vi "Read.Decrypt.7zPayload.vi"(8 "error in (no error)":errorcluster, 9 "Password":string="pw", 10 "File Folder Out":path, 11 "File Path":path) -> (0 "error out":errorcluster)   [LabVIEW 2020, in "PixPack.lvlib"]
uses:
  PixPack.lvlib
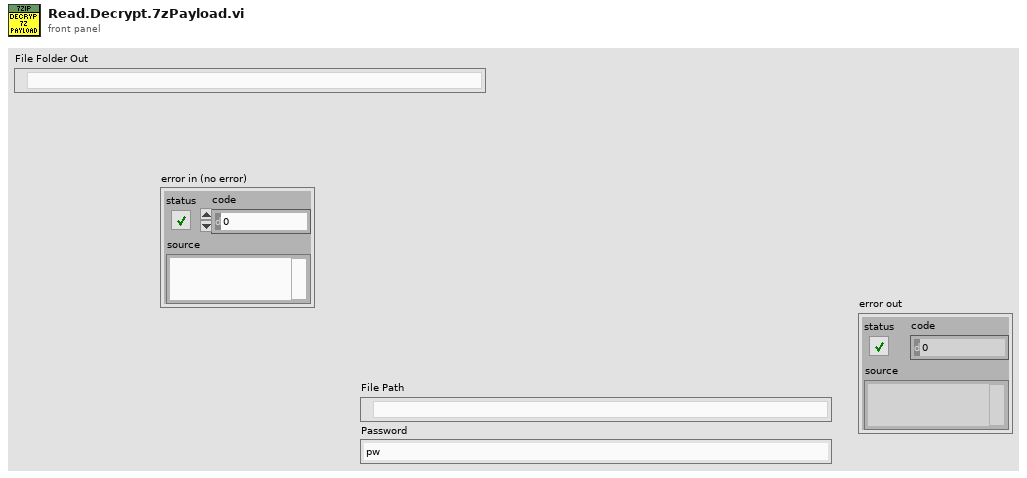
[diagram p1: front panel]
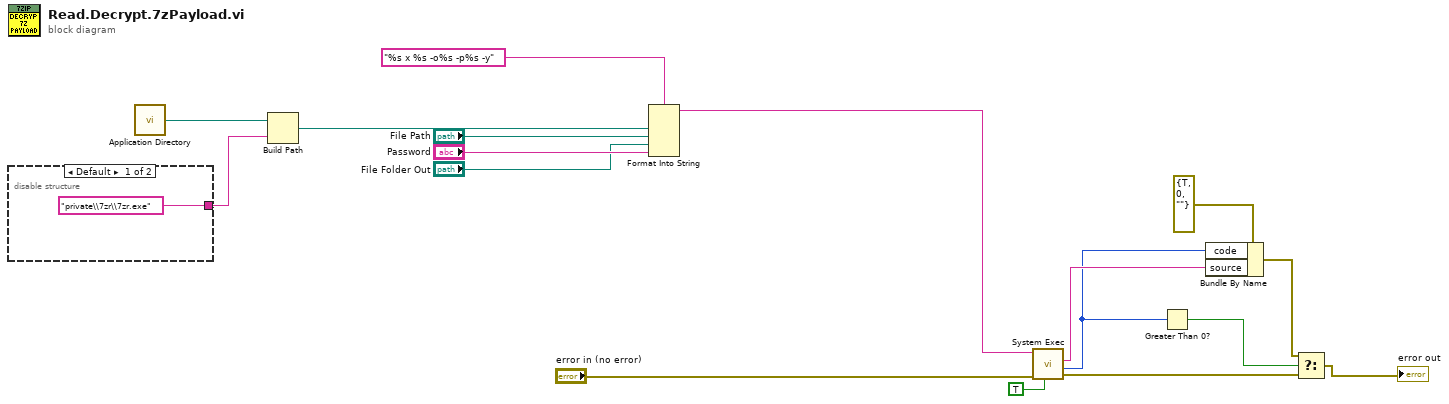
[diagram p0: block diagram]
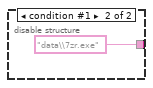
[diagram p2: hidden frame]
diagram:
  n1 = disable-structure shown="Default" {
    disable-tunnel: ["private\\7zr\\7zr.exe" "data\\7zr.exe"] -> w1
    frame condition #0 (active) {
    }
    frame condition #1 {
    }
  }
  n2 = call <vilib>:"Application Directory.vi"() -> ("Application Directory"=w17:path)
  n3 = Build Path(base path=w17, name or relative path=w1) -> (appended path=w13:path)
  n4 = Format Into String(format string="%s x %s -o%s -p%s -y", w13, "File Path", "File Folder Out", "Password") -> (resulting string=w15:string)  [unwired: 2 in, 1 out]
  n5 = call <vilib>:"System Exec.vi"("run minimized? (F)"=TRUE, "error in (no error)"="error in (no error)", "command line"=w15) -> ("error out"=w7:errorcluster, "return code"=w4:i32, "standard error"=w5:string)  [unwired: 5 in, 1 out]
  n6 = Greater Than 0?(x=w4) -> (x > 0?=w8:bool)
  n7 = Bundle By Name(cluster=errorcluster {"status"=TRUE, "code"=0, "source"=""} ("error out"), "code"=w4, "source"=w5) -> (w3:errorcluster)
  n8 = Select(t=w3, s=w8, f=w7) -> (s? t:f=→"error out":errorcluster)
